vi "E07_VariableLocal.vi"() -> ()   [LabVIEW 2026]
panel:
  out "Numeric":dbl
  out "Numeric 2":dbl
  in  "stop":bool
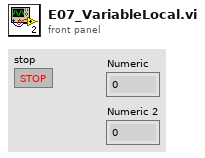
[diagram p1: front panel]
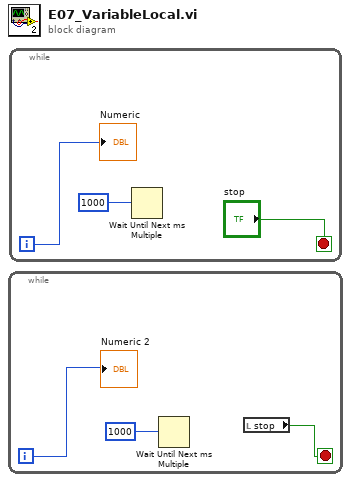
[diagram p0: block diagram]
diagram:
  n1 = while {
    i -> [w2]
    stop <- w1 stop-if-true
    n2 = Wait Until Next ms Multiple(millisecond multiple=u32 1000 ("millisecond timer value")) -> ()  [unwired: 1 out]
    n3 = local read "stop"() -> (w1:bool)
    "Numeric 2" <- w2
  }
  n4 = while {
    i -> [w5]
    stop <- "stop" stop-if-true
    n5 = Wait Until Next ms Multiple(millisecond multiple=u32 1000 ("millisecond timer value")) -> ()  [unwired: 1 out]
    "Numeric" <- w5
  }
